vi "7_Coincidences-JaggedArrayInLabVIEW.vi"() -> ()   [LabVIEW 2015]
uses:
  C:/Users/MX-Microscope/Documents/LabVIEW Data/lvoop_campus_2018/Detector_Class/Swabian/time_tagger_vis/TTCSharp32.dll
  TTCSharp32.dll
panel:
  out "XY Graph":cluster{"Y":dbl[], "Y":dbl[]}[](graph)
  # "The built in test signal (~ 800 to 900 kHz) is applied at different channels at different times to show how to use the class Coincidences"
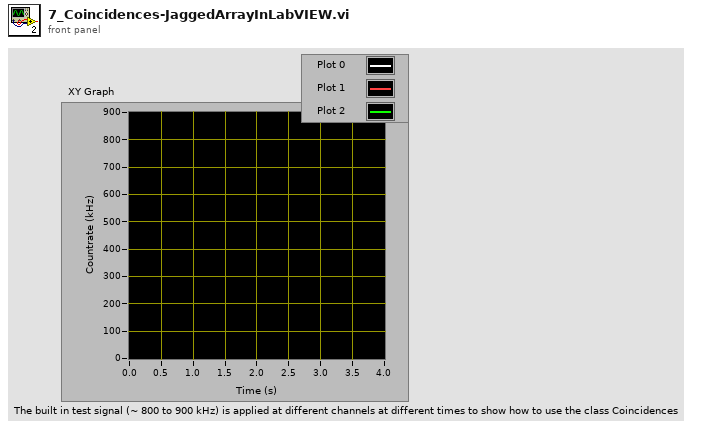
[diagram p1: front panel]
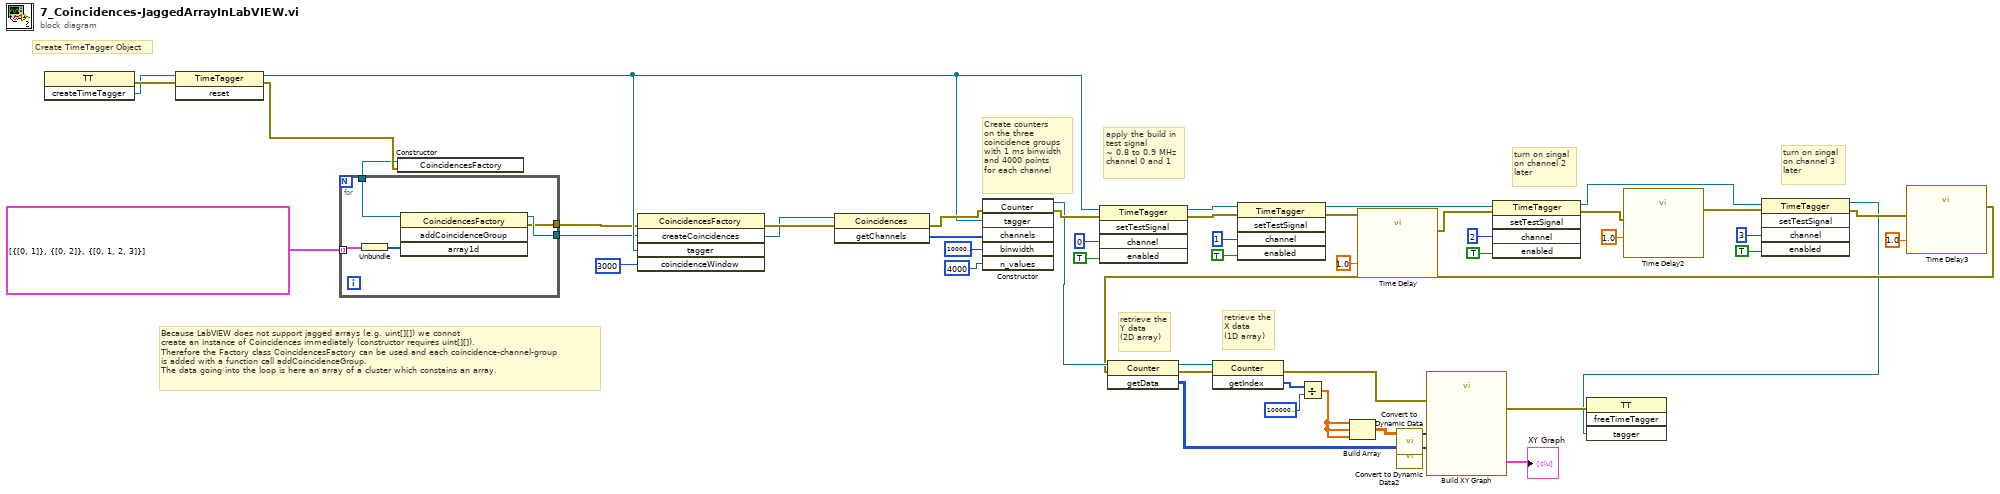
[diagram p0: block diagram]
diagram:
  # "Because LabVIEW does not support jagged arrays (e.g. uint[][]) we connot \ncreate an instance of Coincidences immediately (constructor requires uint[][]).\nTherefore the Factory class CoincidencesFactory can be used and each coincidence-channel-group\nis added with a function call addCoincidenceGroup.\nThe data going into the loop is here an array of a cluster which constains an array."
  # "turn on singal\non channel 3\nlater"
  # "retrieve the\nX data\n(1D array)"
  # "retrieve the\nY data\n(2D array)"
  # "turn on singal\non channel 2\nlater"
  # "apply the build in\ntest signal\n~ 0.8 to 0.9 MHz\nchannel 0 and 1"
  # "Create counters\non the three \ncoincidence groups\nwith 1 ms binwidth\nand 4000 points\nfor each channel"
  # "Create TimeTagger Object"
  n1 = invoke class="TT" method="createTimeTagger"() -> (error out=w47:errorcluster, "createTimeTagger"=w46:refnum<k24>)  [unwired: 3 in, 1 out]
  n2 = invoke class="TimeTagger" method="reset"(reference=w46, error in=w47) -> (reference out=w19:refnum<k24>, error out=w16:errorcluster)  [unwired: 1 in, 1 out]
  n3 = constructor class="CoincidencesFactory"(error in=w16) -> (reference out=w14:refnum<k24>)  [unwired: 2 in, 2 out]
  n4 = for {
    tunnel: cluster{i32[]}[] [{[0, 1]}, {[0, 2]}, {[0, 1, 2, 3]}] -> [w56] mode=indexing
    tunnel: w14 -> [w54]
    tunnel: [w53] -> w13
    tunnel: [w52] -> w12
    n5 = Unbundle(w56) -> (w55:i32[])
    n6 = invoke class="CoincidencesFactory" method="addCoincidenceGroup"(reference=w54, "array1d"=w55) -> (reference out=w53:refnum<k24>, error out=w52:errorcluster)  [unwired: 2 in, 2 out]
  }
  n7 = invoke class="CoincidencesFactory" method="createCoincidences"(reference=w13, error in=w12, "tagger"=w19, "coincidenceWindow"=i64 3000) -> (error out=w18:errorcluster, "createCoincidences"=w17:refnum<k24>)  [unwired: 1 in, 3 out]
  n8 = invoke class="Coincidences" method="getChannels"(reference=w17, error in=w18) -> (error out=w21:errorcluster, "getChannels"=w22:u32[])  [unwired: 1 in, 1 out]
  n9 = constructor class="Counter"(error in=w21, "tagger"=w19, "channels"=w22, "binwidth"=i64 1000000000, "n_values"=4000) -> (reference out=w40:refnum<k24>, error out=w41:errorcluster)  [unwired: 2 in, 5 out]
  n10 = invoke class="TimeTagger" method="setTestSignal"(reference=w19, error in=w41, "channel"=u32 0, "enabled"=TRUE) -> (reference out=w26:refnum<k24>, error out=w25:errorcluster)  [unwired: 1 in, 3 out]
  n11 = invoke class="TimeTagger" method="setTestSignal"(reference=w26, error in=w25, "channel"=u32 1, "enabled"=TRUE) -> (reference out=w24:refnum<k24>, error out=w23:errorcluster)  [unwired: 1 in, 3 out]
  n12 = call "Time Delay"("error in (no error)"=w23, "Delay Time (s)"=1.0) -> ("error out"=w42:errorcluster)  [unwired: 9 in]
  n13 = invoke class="TimeTagger" method="setTestSignal"(reference=w24, error in=w42, "channel"=u32 2, "enabled"=TRUE) -> (reference out=w4:refnum<k24>, error out=w38:errorcluster)  [unwired: 1 in, 3 out]
  n14 = call "Time Delay2"("error in (no error)"=w38, "Delay Time (s)"=1.0) -> ("error out"=w7:errorcluster)  [unwired: 9 in]
  n15 = invoke class="TimeTagger" method="setTestSignal"(reference=w4, error in=w7, "channel"=u32 3, "enabled"=TRUE) -> (reference out=w3:refnum<k24>, error out=w6:errorcluster)  [unwired: 1 in, 3 out]
  n16 = call "Time Delay3"("error in (no error)"=w6, "Delay Time (s)"=1.0) -> ("error out"=w5:errorcluster)  [unwired: 9 in]
  n17 = invoke class="Counter" method="getData"(reference=w40, error in=w5) -> (reference out=w37:refnum<k24>, error out=w36:errorcluster, "getData"=w2:i32[][])  [unwired: 1 in]
  n18 = invoke class="Counter" method="getIndex"(reference=w37, error in=w36) -> (error out=w34:errorcluster, "getIndex"=w31:i64[])  [unwired: 1 in, 1 out]
  n19 = Divide(x=w31, y=i64 1000000000000) -> (x/y=w1:dbl[])
  n20 = Build Array(w1, w1, w1) -> (w33:dbl[][])
  n21 = call "Convert to Dynamic Data"("2D Array"=w33) -> ("Dynamic Data Type"=w32:dynamicdata)  [unwired: 3 in]
  n22 = call "Convert to Dynamic Data2"("2D Array"=w2) -> ("Dynamic Data Type"=w11:dynamicdata)  [unwired: 3 in]
  n23 = call "Build XY Graph"("error in (no error)"=w34, "Y Input"=w11, "X Input"=w32) -> ("error out"=w29:errorcluster, "XY Graph"=→"XY Graph":cluster{"X":dbl[], "Y":dbl[]}[])  [unwired: 7 in]
  n24 = invoke class="TT" method="freeTimeTagger"(error in=w29, "tagger"=w3) -> ()  [unwired: 2 in, 4 out]
